vi "Automotive ECU - Engine Speed.vi"() -> ()   [LabVIEW 2013]
doc: "Sample numeric display item."
uses:
  <vilib>/NI Veristand/Display Template Support/Display Template Support.llb/cluster_Screen Item Settings.ctl
  <vilib>/NI Veristand/Display Template Support/Display Template Support.llb/cluster_Graph Scale Settings.ctl
  <vilib>/NI Veristand/Display Template Support/Display Template Support.llb/cluster_Graph Plot Settings.ctl
  NationalInstruments.VeriStand.SystemStorage
  <vilib>/NI Veristand/Display Template Support/Display Template Support.llb/enum_Display Template Handler Minimal To Widget Msg.ctl
  <vilib>/NI Veristand/Display Template Support/Display Template Support.llb/enum_Display Template Handler Minimal To Workspace.ctl
  Support/Engine Speed Parameters.ctl
  <vilib>/NI Veristand/Execution/Workspace/NI_VS Workspace ExecutionAPI.lvlib
panel:
  in  "Manual Fixed Engine Speed":dbl format="%_5g"
  in  "FIXED \nEngine Speed":T1(radio)
  in  "Min Engine Speed":dbl format="%_5g"
  in  "Manual Desired RPM":dbl format="%_5g"
  in  "Desired RPM":T2(radio)
  out "Engine RPM":dbl(knob) scale=0.0..2400.0 scale format="%#_2f"
  out "Label":string="Numeric"
  in  "NIVS.System Definition Root":refnum<k24>
  in  "NIVS.Gateway IP Address":string
  in  "Item.Data":T3
  # "Min. Engine Speed"
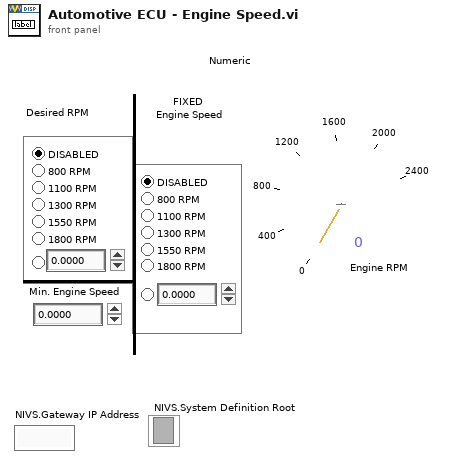
[diagram p1: front panel]
types:
  T1 = enum32{"Radio Selection 1", "Radio Selection 3", "Radio Selection 4", "Radio Selection 5", "Radio Selection 6", "Radio Selection 8", "Radio Selection 7"}
  T2 = enum32{"Radio Selection 1", "Radio Selection 2", "Radio Selection 3", "Radio Selection 4", "Radio Selection 5", "Radio Selection 6", "Radio Selection 7"}
  T3 = typedef "cluster_Screen Item Settings.ctl" = cluster{"Template VI":string, "Position X":i32, "Position Y":i32, "Custom":string, "Show Title Bar":bool, "ID":i32, "Always On Top":bool, "Allow Resize":bool, "Allow Minimize":bool, "Allow Close":bool, "Size to Screen":bool, "Screen.ID":i32, "State":enum16{"Normal", "New"}, "Title":string, "Window Bounds":cluster{"[0]":i16, "[1]":i16, "[2]":i16, "[3]":i16}, "Channel Ref":u64, "Unit":string, "Default Units?":bool, "Flash Limit?":bool, "Color 1":u32, "Color 2":u32, "Color 3":u32, "Color 4":u32, "Bck Color":u32, "Fore Color":u32, "Limit 1":dbl, "Limit 2":dbl, "Limit 3":dbl, "Limit 4":dbl, "Limit Mode 1":i32, "Limit Mode 2":i32, "Limit Mode 3":i32, "Limit Mode 4":i32, "Scale Precision":i32, "Scale Min":dbl, "Scale Max":dbl, "Format":i32, "Precision":i32, "Background Type":i32, "IDs":i32[], "Units":string[], "Labels":string[], "Scale Factor":dbl, "Scale Offset":dbl, "YScale Index":u32[], "XScale":T4, "YScales":T4[], "Plots":T5[], "Update Period":dbl, "History Length":dbl, "My.Ref":refnum<vi>, "Is Control?":bool, "Channel Paths":string[], "Custom Data":variant}
  T4 = typedef "cluster_Graph Scale Settings.ctl" = cluster{"Format":u8, "Precision":u8, "Fit":u8, "Label":string, "Use Default Label":bool, "Label Visible":bool, "Min":dbl, "Max":dbl}
  T5 = typedef "cluster_Graph Plot Settings.ctl" = cluster{"Bar Style":u8, "Fill To":i16, "Fill/PtColor":u32, "Line Style":u8, "Line Width":u8, "Color":u32, "Interp":u8, "Point Style":u8}
  T6 = typedef "enum_Display Template Handler Minimal To Workspace.ctl" = cluster{"Operation":enum16{"SetCustomData", "DeleteItem"}, "Data":variant}
  T7 = typedef "enum_Display Template Handler Minimal To Widget Msg.ctl" = enum16{"Stop", "LaunchConfigDialog"}
  T8 = typedef "Engine Speed Parameters.ctl" = cluster{"Initialized?":bool, "Desired RPM":dbl, "Fixed Engine Speed":dbl, "Min Engine Speed":dbl, "Two Bindings? ":bool, "Dial Shows Fixed?":bool, "Top Pane Color":u32, "Left Pane Color":u32, "Right Pane Color":u32, "Label":string, "Fixed Path":cluster{"NodePathArray":string[], "Node Path":string}, "Desired Path":cluster{"NodePathArray":string[], "Node Path":string}, "Default Control Values":variant[], "Dial Max RPM":dbl}
  T9 = typedef "NI_VS Workspace ExecutionAPI.lvlib/WorkspaceAPI.ctl" = refnum<k24>
  T10 = enum8{"Enabled", "Disabled", "Disabled and Grayed Out"}
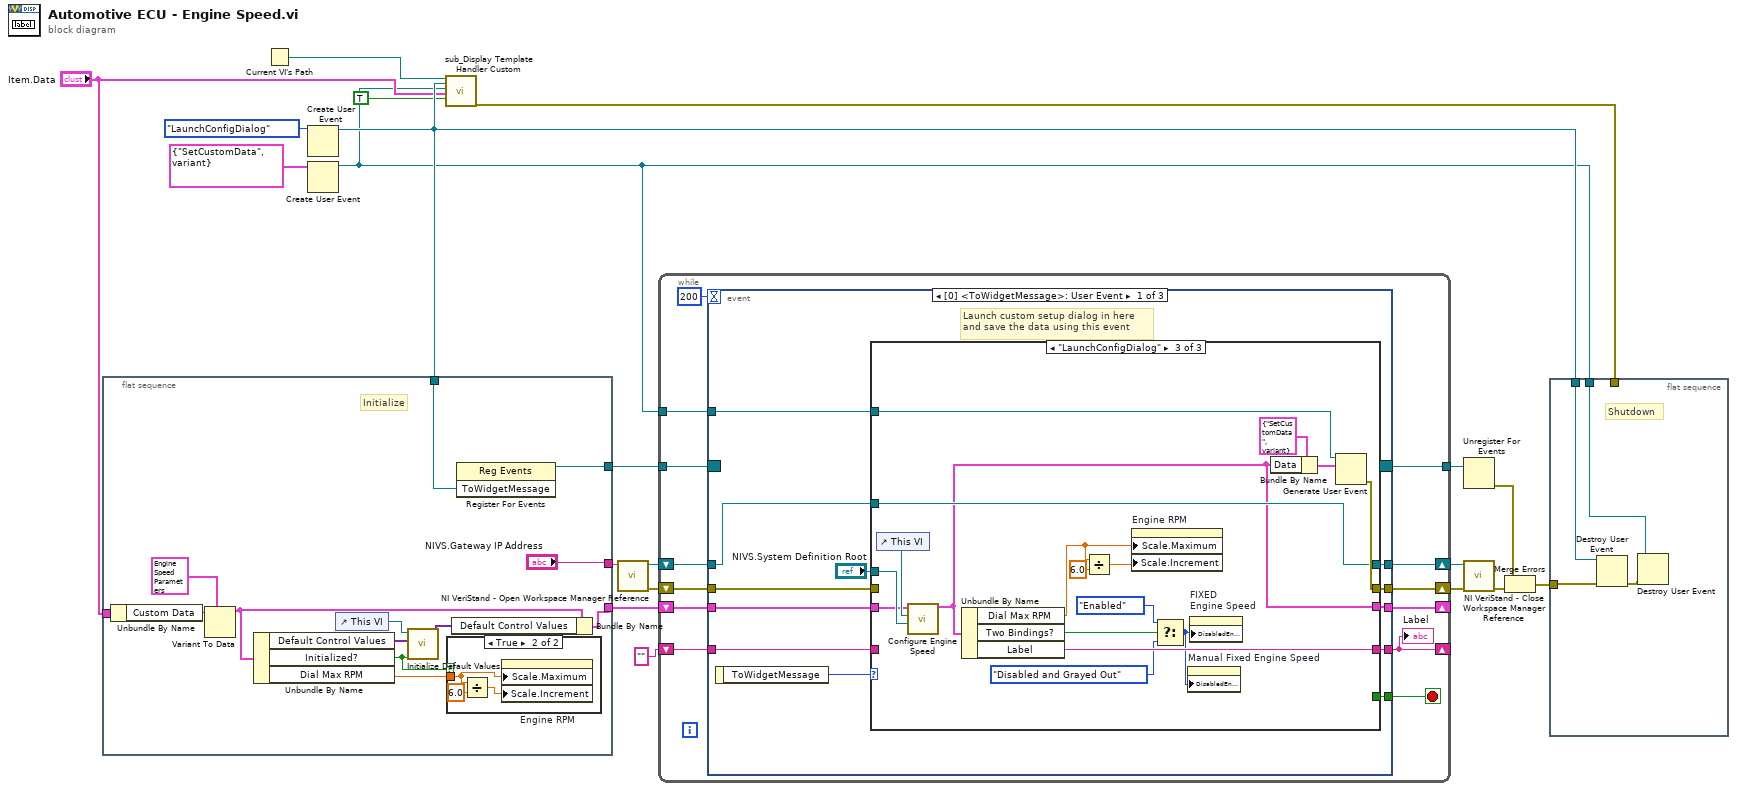
[diagram p0: block diagram]
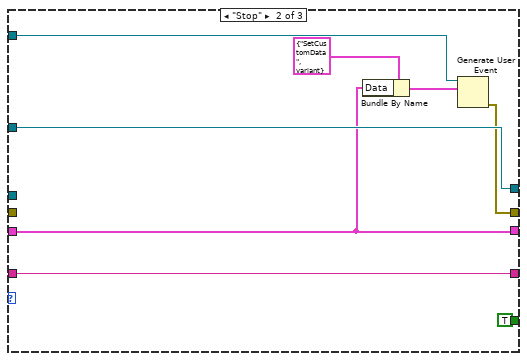
[diagram p4: hidden frame]
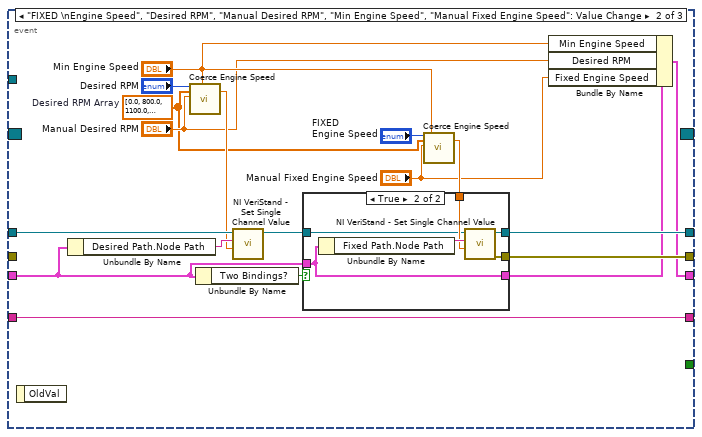
[diagram p5: hidden frame]
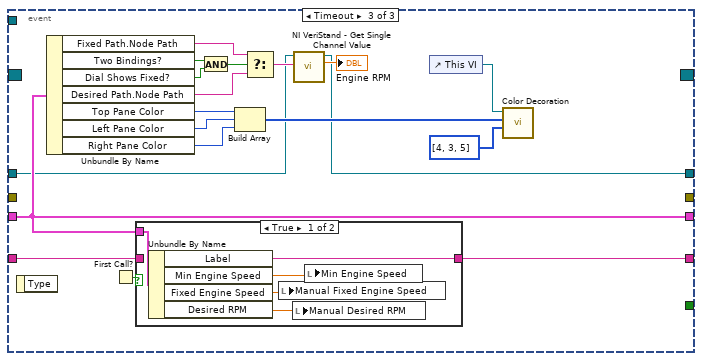
[diagram p7: hidden frame]
diagram:
  n1 = flat-sequence {
    tunnel: [w33] -> w18
    tunnel: w15 -> [w32]
    tunnel: "Item.Data" -> [w31]
    tunnel: [w24] -> w9
    tunnel: ["NIVS.Gateway IP Address"] -> w4
    frame #0 {
      # "Initialize"
      n2 = Unbundle By Name(w31) -> ("Custom Data"=w30:variant)
      n3 = Variant To Data(type=T8 {"Initialized?"=FALSE, "Desired RPM"=0.0, "Fixed Engine Speed"=0.0, "Min Engine Speed"=0.0, "Two Bindings? "=FALSE, "Dial Shows Fixed?"=FALSE, "Top Pane Color"=0, "Left Pane Color"=0, "Right Pane Color"=0, "Label"="", "Fixed Path"={"NodePathArray"=[], "Node Path"=""}, "Desired Path"={"NodePathArray"=[], "Node Path"=""}, "Default Control Values"=[], "Dial Max RPM"=0.0} ("Slide Parameters"), Variant=w30) -> (data=w23:T8)  [unwired: 1 in, 1 out]
      n4 = Unbundle By Name(w23) -> ("Default Control Values"=w26:variant[], "Initialized?"=w21:bool, "Dial Max RPM"=w22:dbl)
      n5 = control-ref of="This VI"() -> (w25:refnum<vi>)
      n6 = call "Initialize Default Values.vi"("Initialized?"=w21, "Default Control Values in"=w26, "VI in"=w25) -> ("Default Control Values out"=w27:variant[])  [unwired: 7 in, 1 out]
      n7 = case shown="True" w21 {
        tunnel: w22 -> [_ w36]
        frame False {
        }
        frame True {
          n8 = Divide(x=w36, y=6.0) -> (x/y=w34:dbl)
          n9 = property on="Engine RPM" class="Knob (strict)"("Scale.Maximum"=w36, "Scale.Increment"=w34) -> ()  [unwired: 2 in, 2 out]
        }
      }
      n10 = Bundle By Name(cluster=w23, "Default Control Values"=w27) -> (w24:T8)
      n11 = register-events(w32) -> (reference out=w33:refnum<event-registration>)  [unwired: 2 in, 1 out]
    }
  }
  n12 = Current VI's Path() -> (path=w13:path)
  n13 = Create User Event(user event datatype=enum_Display_Template_Handler_Minimal_To_Widget_Msg."LaunchConfigDialog" ("ToWidgetMessage")) -> (user event=w15:refnum<user-event>)  [unwired: 1 in, 1 out]
  n14 = Create User Event(user event datatype=T6 {"Operation"=enum."SetCustomData", "Data"=variant} ("Data")) -> (user event=w11:refnum<user-event>)  [unwired: 1 in, 1 out]
  n15 = call <vilib>:"sub_Display Template Handler Custom.vi"("Parent.Path"=w13, "ToWidgetEvent"=w15, "ToWorkspace"=w11, "Item.Data"="Item.Data", "Resizable"=TRUE) -> ("error out"=w20:errorcluster)  [unwired: 14 in]
  n16 = call <vilib>:"NI VeriStand - Open Workspace Manager Reference.vi"("Gateway IP Address (\"\": localhost)"=w4) -> ("error out"=w7:errorcluster, "WorkspaceManager"=w8:T9)  [unwired: 9 in]
  n17 = while {
    tunnel: w18 -> [w49]
    tunnel: [w47] -> w17
    tunnel: w11 -> [w46]
    shift-right: [w38] -> _
    shift-left: w9 -> [w45]
    shift-right: [w42] -> w6
    shift-left: w8 -> [w44]
    shift-right: [w39] -> w5
    shift-left: w7 -> [w43]
    shift-right: [w40] -> _
    shift-left: "" ("Out") -> [w41]
    stop <- w48 stop-if-true
    n18 = event shown="[0] <ToWidgetMessage>: User Event" {
      selector: w49 -> [_ _ _]
      dyn-events: [_ _ _] -> w47
      timeout: 200 -> [_ _ _]
      tunnel: [w60 _ _] -> w48
      tunnel: w46 -> [w59 _ _]
      tunnel: w45 -> [w55 w98 w130]
      tunnel: w44 -> [w58 w100 w121]
      tunnel: w43 -> [w53 _ _]
      tunnel: [w57 w106 w120] -> w42
      tunnel: [w52 w105 _] -> w39
      tunnel: [w51 w108 w134] -> w40
      tunnel: w41 -> [w50 w108 w133]
      tunnel: [w54 w96 w130] -> w38
      event User Event {
        # "Launch custom setup dialog in here\nand save the data using this event"
        n19 = event-data() -> ("ToWidgetMessage"=w61:T7)  [unwired: 1 out]
        n20 = case shown="\"LaunchConfigDialog\"" w61 {
          tunnel: [_ TRUE _] -> w60
          tunnel: w59 -> [_ w69 w88]
          tunnel: w58 -> [w65 w72 w83]
          tunnel: [w65 w72 w83] -> w57
          tunnel: "NIVS.System Definition Root" -> [_ _ w86]
          tunnel: w55 -> [w64 w68 w81]
          tunnel: [w64 w68 w82] -> w54
          tunnel: w53 -> [w62 _ _]
          tunnel: [w62 w67 w87] -> w52
          tunnel: [w63 w66 w84] -> w51
          tunnel: w50 -> [w63 w66 _]
          frame Default {
          }
          frame "Stop" {
            n21 = Bundle By Name(cluster=T6 {"Operation"=enum."SetCustomData", "Data"=variant} ("event data"), "Data"=w68) -> (w70:T6)
            n22 = Generate User Event(user event=w69, event data cluster=w70) -> (error out=w67:errorcluster)  [unwired: 2 in, 1 out]
          }
          frame "LaunchConfigDialog" {
            n23 = control-ref of="This VI"() -> (w85:refnum<vi>)
            n24 = call "Configure Engine Speed.vi"("NIVS.System Definition Root"=w86, "VI Reference"=w85, "Engine Speed Parameters in"=w81) -> ("Engine Speed Parameters out"=w82:T8)  [unwired: 7 in, 1 out]
            n25 = Unbundle By Name(w82) -> ("Dial Max RPM"=w74:dbl, "Two Bindings?"=w79:bool, "Label"=w84:string)
            n26 = Divide(x=w74, y=6.0) -> (x/y=w75:dbl)
            n27 = property on="Engine RPM" class="Knob (strict)"("Scale.Maximum"=w74, "Scale.Increment"=w75) -> ()  [unwired: 2 in, 2 out]
            n28 = Select(t=T10."Enabled" ("Disabled"), s=w79, f=T10."Disabled and Grayed Out" ("Disabled")) -> (s? t:f=w77:T10)
            n29 = property on="Manual Fixed Engine Speed" class="DigNum (strict)"("DisabledEnum"=w77) -> ()  [unwired: 2 in, 2 out]
            n30 = property on="FIXED \nEngine Speed" class="RadioBtnsControl (strict)"("DisabledEnum"=w77) -> ()  [unwired: 2 in, 2 out]
            n31 = Bundle By Name(cluster=T6 {"Operation"=enum."SetCustomData", "Data"=variant} ("event data"), "Data"=w82) -> (w90:T6)
            n32 = Generate User Event(user event=w88, event data cluster=w90) -> (error out=w87:errorcluster)  [unwired: 2 in, 1 out]
          }
        }
      }
      event "FIXED \nEngine Speed", "Desired RPM", "Manual Desired RPM", "Min Engine Speed", "Manual Fixed Engine Speed": Value Change {
        w91 = dbl[] [0.0, 800.0, 1100.0, 1300.0, 1550.0, 1800.0, 0.0]  # Desired RPM Array
        n33 = event-data() -> ()  [unwired: 2 out]
        n34 = Unbundle By Name(w98) -> ("Desired Path.Node Path"=w101:string)
        n35 = call "Coerce Engine Speed.vi"("RPM Selection In"="Desired RPM", "RPM Array"=w91, "Manual Desired RPM"="Manual Desired RPM", "Min Engine Speed in"="Min Engine Speed") -> ("Min Engine Speed out"=w97:dbl)  [unwired: 15 in]
        n36 = Unbundle By Name(w98) -> ("Two Bindings?"=w107:bool)
        n37 = call <vilib>:"NI VeriStand - Set Single Channel Value.vi"("Value"=w97, "Channel"=w101, "WorkspaceManager in"=w100) -> ("WorkspaceManager out"=w99:T9)  [unwired: 7 in, 1 out]
        n38 = call "Coerce Engine Speed.vi"("RPM Selection In"="FIXED \nEngine Speed", "RPM Array"=w91, "Manual Desired RPM"="Manual Fixed Engine Speed", "Min Engine Speed in"="Min Engine Speed") -> ("Min Engine Speed out"=w102:dbl)  [unwired: 15 in]
        n39 = case shown="True" w107 {
          tunnel: w99 -> [w109 w111]
          tunnel: w98 -> [w110 w116]
          tunnel: [w109 w114] -> w106
          tunnel: [_ w115] -> w105
          tunnel: [w110 w116] -> w95
          tunnel: w102 -> [_ w112]
          frame False {
          }
          frame True {
            n40 = Unbundle By Name(w116) -> ("Fixed Path.Node Path"=w113:string)
            n41 = call <vilib>:"NI VeriStand - Set Single Channel Value.vi"("Value"=w112, "Channel"=w113, "WorkspaceManager in"=w111) -> ("error out"=w115:errorcluster, "WorkspaceManager out"=w114:T9)  [unwired: 7 in]
          }
        }
        n42 = Bundle By Name(cluster=w95, "Min Engine Speed"="Min Engine Speed", "Desired RPM"="Manual Desired RPM", "Fixed Engine Speed"="Manual Fixed Engine Speed") -> (w96:T8)
      }
      event Timeout {
        n43 = event-data() -> ()  [unwired: 2 out]
        n44 = Unbundle By Name(w130) -> ("Fixed Path.Node Path"=w125:string, "Two Bindings?"=w128:bool, "Dial Shows Fixed?"=w127:bool, "Desired Path.Node Path"=w124:string, "Top Pane Color"=w129:u32, "Left Pane Color"=w118:u32, "Right Pane Color"=w117:u32)
        n45 = First Call?() -> (First Call?: T/F=w135:bool)
        n46 = case shown="True" w135 {
          tunnel: w133 -> [_ w141]
          tunnel: [w139 w141] -> w134
          tunnel: w130 -> [w140 _]
          frame True {
            n47 = Unbundle By Name(w140) -> ("Label"=w139:string, "Min Engine Speed"=w136:dbl, "Fixed Engine Speed"=w137:dbl, "Desired RPM"=w138:dbl)
            n48 = local write "Manual Fixed Engine Speed"(w137) -> ()
            n49 = local write "Manual Desired RPM"(w138) -> ()
            n50 = local write "Min Engine Speed"(w136) -> ()
          }
          frame False {
            # "If this is the first call, update label"
          }
        }
        n51 = And(x=w128, y=w127) -> (x .and. y?=w126:bool)
        n52 = Build Array(w129, w118, w117) -> (w131:u32[])
        n53 = Select(t=w125, s=w126, f=w124) -> (s? t:f=w123:string)
        n54 = call <vilib>:"NI VeriStand - Get Single Channel Value.vi"("Channel"=w123, "WorkspaceManager in"=w121) -> ("Value"=→"Engine RPM":dbl, "WorkspaceManager out"=w120:T9)  [unwired: 7 in, 1 out]
        n55 = control-ref of="This VI"() -> (w132:refnum<vi>)
        n56 = call "Color Decoration.vi"("VI reference"=w132, "Color Array"=w131, "Index Array"=u32[] [4, 3, 5] ("Color Array")) -> ()  [unwired: 7 in, 1 out]
      }
    }
    "Label" <- w40
  }
  n57 = Unregister For Events(event registration refnum=w17) -> (error out=w16:errorcluster)  [unwired: 1 in]
  n58 = call <vilib>:"NI VeriStand - Close Workspace Manager Reference.vi"("error in (no error)"=w5, "WorkspaceManager"=w6) -> ("error out"=w1:errorcluster)  [unwired: 9 in]
  n59 = Merge Errors(w16, w1) -> (w2:errorcluster)
  n60 = flat-sequence {
    tunnel: w20 -> [_]
    tunnel: w2 -> [w144]
    tunnel: w15 -> [w145]
    tunnel: w11 -> [w142]
    frame #0 {
      # "Shutdown"
      n61 = Destroy User Event(user event=w145, error in=w144) -> (error out=w143:errorcluster)
      n62 = Destroy User Event(user event=w142, error in=w143) -> ()  [unwired: 1 out]
    }
  }
